vi "tempconfigAO.vi"(1 "Temp Config in":T1, 2 "command":string) -> (0 "Temp Config out":T1)   [LabVIEW 2015]
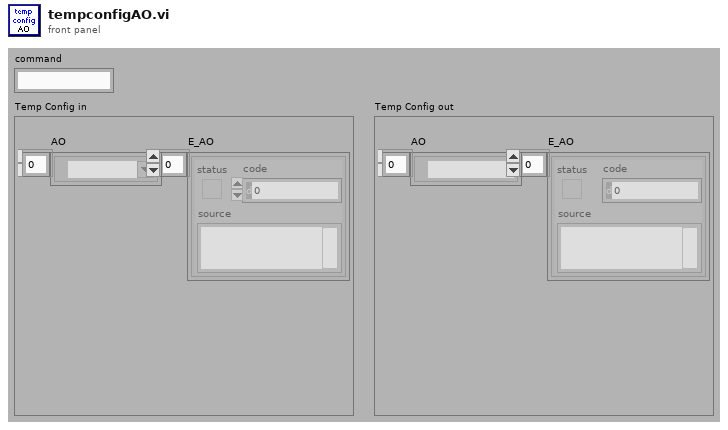
[diagram p1: front panel]
types:
  T1 = cluster{"AO":refnum<k21>[], "E_AO":errorcluster[]}
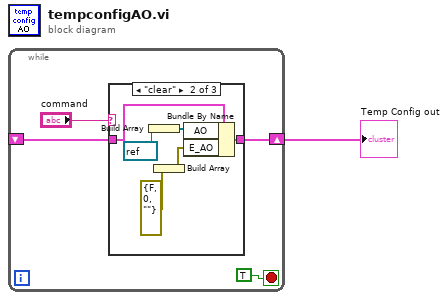
[diagram p0: block diagram]
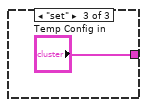
[diagram p3: hidden frame]
diagram:
  n1 = while {
    shift-right: [w3] -> w1
    shift-left: _ -> [w2]
    stop <- TRUE stop-if-true
    n2 = case shown="\"clear\"" "command" {
      tunnel: [w6 w9 "Temp Config in"] -> w3
      tunnel: w2 -> [w6 w12 _]
      frame "get", Default {
      }
      frame "clear" {
        n3 = Build Array(refnum<k21> refnum ("XY")) -> (w7:refnum<k21>[])
        n4 = Build Array(errorcluster {"status"=FALSE, "code"=0, "source"=""} ("E_AI")) -> (w8:errorcluster[])
        n5 = Bundle By Name(cluster=w12, "AO"=w7, "E_AO"=w8) -> (w9:T1)
      }
      frame "set" {
      }
    }
  }
  "Temp Config out" <- w1
